vi "ziVectorWrite.vi"(3 "error in":errorcluster, 4 "VectorWave In":T1, 5 "Path":string, 6 "Handle in":T2 {"Handle" format="0x%08x"; "Conn" format="0x%08x"}) -> (0 "error out":errorcluster, 1 "VectorWave Out":T1, 2 "Handle out":T2 {"Handle" format="0x%08x"; "Conn" format="0x%08x"})   [LabVIEW 2019, in "Zurich Instruments LabOne.lvlib"]
doc: "This vi retrieves the numerical value of the specified node as an double-type value. The vi returns the value first found that matches Path if more than one value is available (a wildcard is used in the Path)."
uses:
  Zurich Instruments LabOne.lvlib
  ziTypeHandle.ctl
  Data/ziTypeCoreVectorWave.ctl
  Private/ziLV64.dll
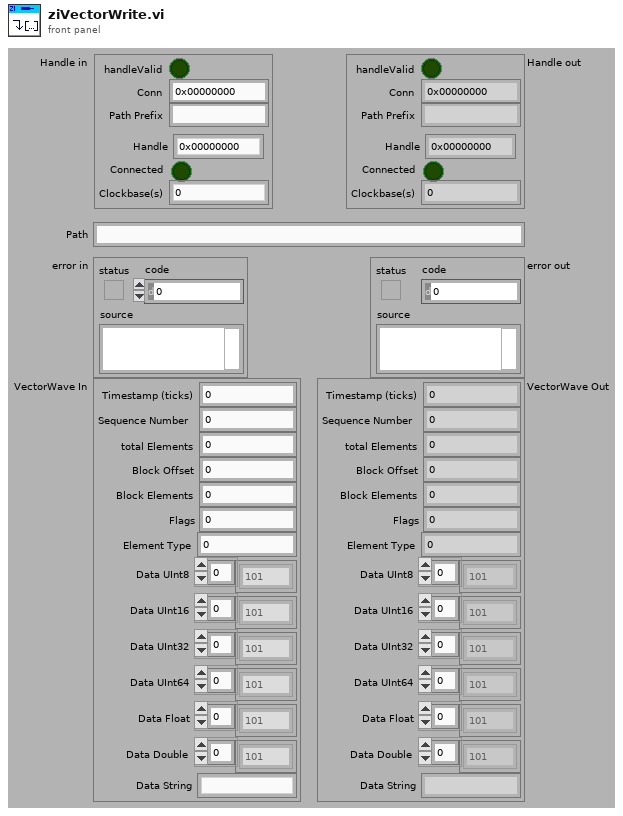
[diagram p1: front panel]
types:
  T1 = typedef "Zurich Instruments LabOne.lvlib/ziTypeCoreVectorWave.ctl" = cluster{"Timestamp (ticks)":u64, "Sequence Number":u32, "total Elements":u64, "Block Offset":u64, "Block Elements":u32, "Flags":u8, "Element Type":u8, "Data UInt8":u8[], "Data UInt16":u16[], "Data UInt32":u32[], "Data UInt64":u64[], "Data Float":sgl[], "Data Double":dbl[], "Data String":string}
  T2 = typedef "Zurich Instruments LabOne.lvlib/ziTypeHandle.ctl" = cluster{"handleValid":bool, "Conn":u64, "Path Prefix":string, "Handle":u64, "Connected":bool, "Clockbase(s)":dbl}
  T3 = enum8{"Unit8", "Unit16", "Unit32", "Unit64", "Float", "Double", "ASCII", "NA"}
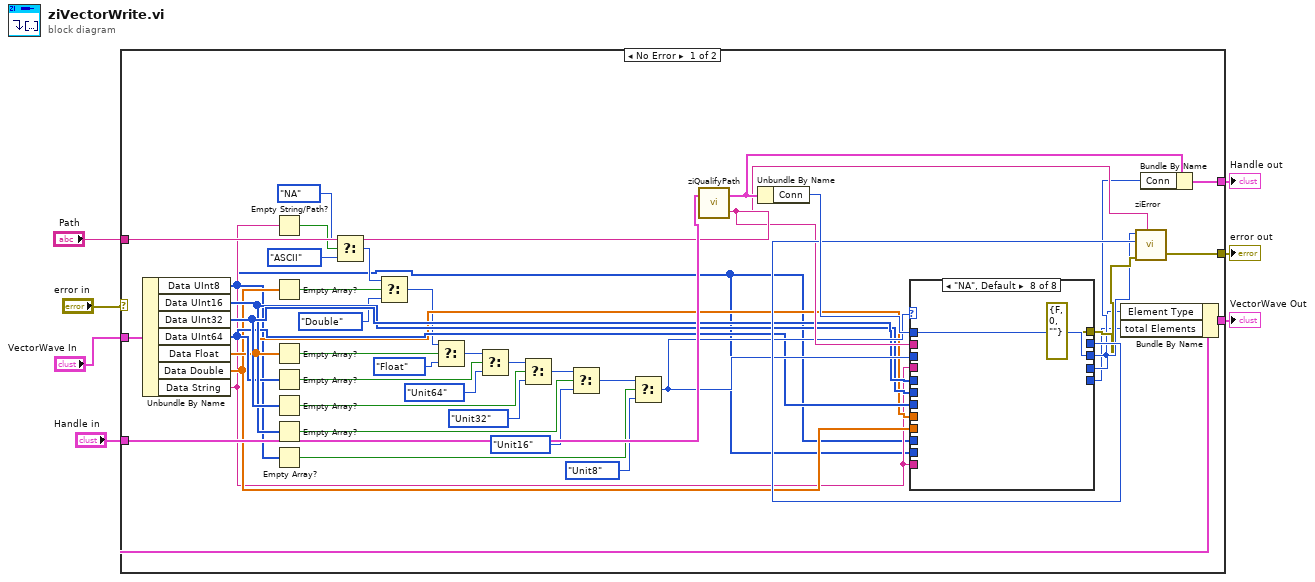
[diagram p0: block diagram]
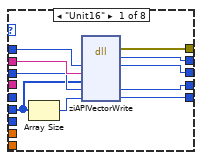
[diagram p2: hidden frame]
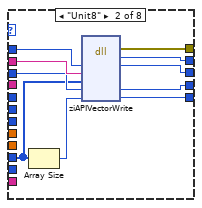
[diagram p3: hidden frame]
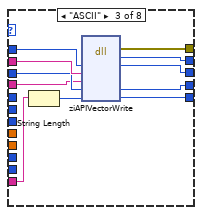
[diagram p4: hidden frame]
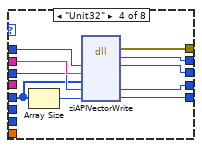
[diagram p5: hidden frame]
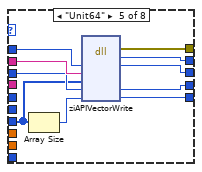
[diagram p6: hidden frame]
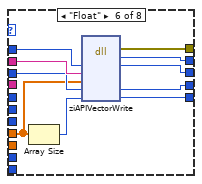
[diagram p7: hidden frame]
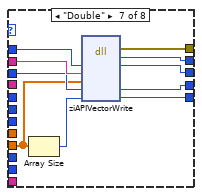
[diagram p8: hidden frame]
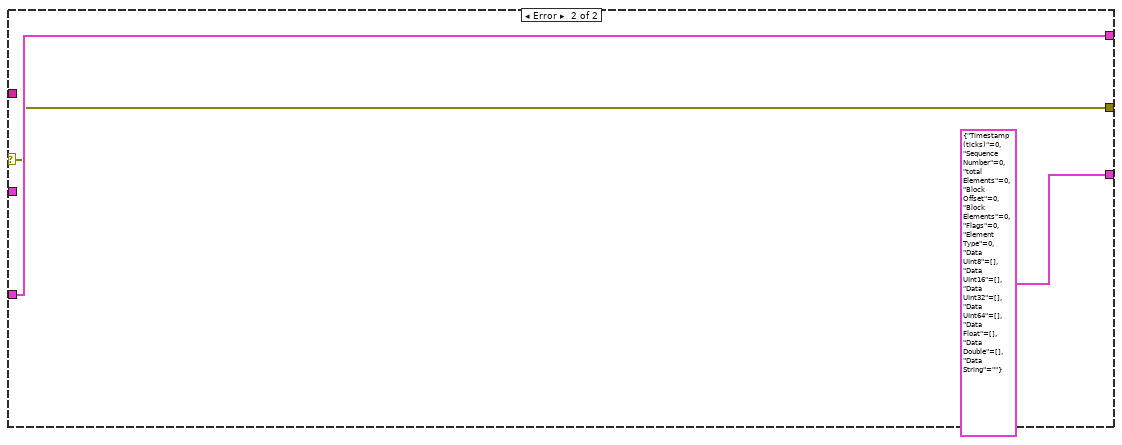
[diagram p9: hidden frame]
diagram:
  n1 = case shown="No Error" "error in" {
    selector: "error in" -> [_ w125]
    tunnel: [w50 w125] -> w7
    tunnel: [w49 w126] -> w6
    tunnel: "Handle in" -> [w48 w126]
    tunnel: "Path" -> [w47 _]
    tunnel: "VectorWave In" -> [w33 _]
    tunnel: [w32 T1 {"Timestamp (ticks)"=0, "Sequence Number"=0, "total Elements"=0, "Block Offset"=0, "Block Elements"=0, "Flags"=0, "Element Type"=0, "Data UInt8"=[], "Data UInt16"=[], "Data UInt32"=[], "Data UInt64"=[], "Data Float"=[], "Data Double"=[], "Data String"=""} ("VectorWave In")] -> w2
    frame No Error {
      n2 = Unbundle By Name(w33) -> ("Data UInt8"=w8:u8[], "Data UInt16"=w27:u16[], "Data UInt32"=w28:u32[], "Data UInt64"=w26:u64[], "Data Float"=w25:sgl[], "Data Double"=w24:dbl[], "Data String"=w23:string)
      n3 = Empty String/Path?(string/path=w23) -> (empty?=w46:bool)
      n4 = Empty Array?(array=w24) -> (empty?=w45:bool)
      n5 = Empty Array?(array=w25) -> (empty?=w44:bool)
      n6 = Empty Array?(array=w26) -> (empty?=w43:bool)
      n7 = Empty Array?(array=w28) -> (empty?=w42:bool)
      n8 = Empty Array?(array=w27) -> (empty?=w41:bool)
      n9 = Empty Array?(array=w8) -> (empty?=w40:bool)
      n10 = Select(t=T3."NA", s=w46, f=T3."ASCII") -> (s? t:f=w9:T3)
      n11 = Select(t=w9, s=w45, f=T3."Double") -> (s? t:f=w10:T3)
      n12 = Select(t=w10, s=w44, f=T3."Float") -> (s? t:f=w11:T3)
      n13 = Select(t=w11, s=w43, f=T3."Unit64") -> (s? t:f=w12:T3)
      n14 = Select(t=w12, s=w42, f=T3."Unit32") -> (s? t:f=w13:T3)
      n15 = Select(t=w13, s=w41, f=T3."Unit16") -> (s? t:f=w14:T3)
      n16 = Select(t=w14, s=w40, f=T3."Unit8") -> (s? t:f=w29:T3)
      n17 = call "ziQualifyPath.vi"("Path In"=w47, "Handle In"=w48) -> ("Path Out"=w35:string, "Handle Out"=w36:T2)
      n18 = Unbundle By Name(w36) -> ("Conn"=w39:u64)
      n19 = case shown="\"NA\", Default" w29 {
        tunnel: w39 -> [w60 w70 w81 w91 w101 w111 w121 w123]
        tunnel: [w59 w69 w80 w90 w100 w110 w120 _] -> w38
        tunnel: [w58 w68 w79 w89 w99 w109 w119 errorcluster {"status"=FALSE, "code"=0, "source"=""} ("error out")] -> w37
        tunnel: w35 -> [w57 w67 w78 w88 w98 w108 w118 _]
        tunnel: [w56 w66 w77 w87 w97 w107 w117 w123] -> w34
        tunnel: w29 -> [w54 w64 w76 w85 w95 w105 w115 _]
        tunnel: [w53 w63 w75 w84 w94 w104 w114 _] -> w31
        tunnel: [w52 w62 w74 w83 w93 w103 w113 _] -> w30
        tunnel: w28 -> [_ _ _ w82 _ _ _ _]
        tunnel: w27 -> [w51 _ _ _ _ _ _ _]
        tunnel: w26 -> [_ _ _ _ w92 _ _ _]
        tunnel: w25 -> [_ _ _ _ _ w102 _ _]
        tunnel: w24 -> [_ _ _ _ _ _ w112 _]
        tunnel: w23 -> [_ _ w71 _ _ _ _ _]
        tunnel: w23 -> [_ _ w73 _ _ _ _ _]
        tunnel: w8 -> [_ _ _ _ _ _ _ _]
        tunnel: w8 -> [_ w61 _ _ _ _ _ _]
        frame "Unit16" {
          n20 = Array Size(array=w51) -> (size(s)=w55:i32)
          n21 = dll-call lib="G:/01_software/CryoTUM/sub_vi-s/Equipment/Zurich Instruments LabOne/Private/ziLV*.*" fn="ziAPIVectorWrite"("Conn"=w60, "Path"=w57, "Pointer"=w51, "vectorElementType"=w54, "vectorSizeElements"=w55) -> (error out=w58:errorcluster, "return type"=w59:u8, "Conn"=w56:u64, "vectorElementType"=w53:u8, "vectorSizeElements"=w52:u64)  [unwired: 3 in, 3 out]
        }
        frame "Unit8" {
          n22 = Array Size(array=w61) -> (size(s)=w65:i32)
          n23 = dll-call lib="G:/01_software/CryoTUM/sub_vi-s/Equipment/Zurich Instruments LabOne/Private/ziLV*.*" fn="ziAPIVectorWrite"("Conn"=w70, "Path"=w67, "Pointer"=w61, "vectorElementType"=w64, "vectorSizeElements"=w65) -> (error out=w68:errorcluster, "return type"=w69:u8, "Conn"=w66:u64, "vectorElementType"=w63:u8, "vectorSizeElements"=w62:u64)  [unwired: 3 in, 3 out]
        }
        frame "ASCII" {
          n24 = String Length(string=w71) -> (length=w72:i32)
          n25 = dll-call lib="G:/01_software/CryoTUM/sub_vi-s/Equipment/Zurich Instruments LabOne/Private/ziLV*.*" fn="ziAPIVectorWrite"("Conn"=w81, "Path"=w78, "Pointer"=w73, "vectorElementType"=w76, "vectorSizeElements"=w72) -> (error out=w79:errorcluster, "return type"=w80:u8, "Conn"=w77:u64, "vectorElementType"=w75:u8, "vectorSizeElements"=w74:u64)  [unwired: 3 in, 3 out]
        }
        frame "Unit32" {
          n26 = Array Size(array=w82) -> (size(s)=w86:i32)
          n27 = dll-call lib="G:/01_software/CryoTUM/sub_vi-s/Equipment/Zurich Instruments LabOne/Private/ziLV*.*" fn="ziAPIVectorWrite"("Conn"=w91, "Path"=w88, "Pointer"=w82, "vectorElementType"=w85, "vectorSizeElements"=w86) -> (error out=w89:errorcluster, "return type"=w90:u8, "Conn"=w87:u64, "vectorElementType"=w84:u8, "vectorSizeElements"=w83:u64)  [unwired: 3 in, 3 out]
        }
        frame "Unit64" {
          n28 = Array Size(array=w92) -> (size(s)=w96:i32)
          n29 = dll-call lib="G:/01_software/CryoTUM/sub_vi-s/Equipment/Zurich Instruments LabOne/Private/ziLV*.*" fn="ziAPIVectorWrite"("Conn"=w101, "Path"=w98, "Pointer"=w92, "vectorElementType"=w95, "vectorSizeElements"=w96) -> (error out=w99:errorcluster, "return type"=w100:u8, "Conn"=w97:u64, "vectorElementType"=w94:u8, "vectorSizeElements"=w93:u64)  [unwired: 3 in, 3 out]
        }
        frame "Float" {
          n30 = Array Size(array=w102) -> (size(s)=w106:i32)
          n31 = dll-call lib="G:/01_software/CryoTUM/sub_vi-s/Equipment/Zurich Instruments LabOne/Private/ziLV*.*" fn="ziAPIVectorWrite"("Conn"=w111, "Path"=w108, "Pointer"=w102, "vectorElementType"=w105, "vectorSizeElements"=w106) -> (error out=w109:errorcluster, "return type"=w110:u8, "Conn"=w107:u64, "vectorElementType"=w104:u8, "vectorSizeElements"=w103:u64)  [unwired: 3 in, 3 out]
        }
        frame "Double" {
          n32 = Array Size(array=w112) -> (size(s)=w116:i32)
          n33 = dll-call lib="G:/01_software/CryoTUM/sub_vi-s/Equipment/Zurich Instruments LabOne/Private/ziLV*.*" fn="ziAPIVectorWrite"("Conn"=w121, "Path"=w118, "Pointer"=w112, "vectorElementType"=w115, "vectorSizeElements"=w116) -> (error out=w119:errorcluster, "return type"=w120:u8, "Conn"=w117:u64, "vectorElementType"=w114:u8, "vectorSizeElements"=w113:u64)  [unwired: 3 in, 3 out]
        }
        frame "NA", Default {
        }
      }
      n34 = Bundle By Name(cluster=w33, "Element Type"=w31, "total Elements"=w30) -> (w32:T1)
      n35 = call "ziError.vi"("Conn"=w34, "ziErrorCode"=w38, "Error In"=w37, "Annotation"=w35) -> ("Error Out"=w50:errorcluster)  [unwired: 1 in, 1 out]
      n36 = Bundle By Name(cluster=w36, "Conn"=w34) -> (w49:T2)
    }
    frame Error {
    }
  }
  "Handle out" <- w6
  "error out" <- w7
  "VectorWave Out" <- w2
